vi "Result.vi"(8 "error in (no error)":errorcluster, 10 "Result":T1={"Case"="", "Message"="", "Description"="", "Status"=enum."Passed", "Result Type"=enum."Case", "Execution Time"=0.0}, 11 "Test Result Tree V2 in":refnum<class "Test Result Tree V2.lvclass">) -> (0 "error out":errorcluster, 3 "Test Result Tree V2 out":refnum<class "Test Result Tree V2.lvclass">)   [LabVIEW 2020, in "Test Result Tree V2.lvclass"]
uses:
  Test Result Tree V2.lvclass
  C:/Git/astemes-lunit/source/Framework/Helper Classes/Test Tree/Test Tree.lvclass
  Result/Result.ctl
  Result/Status.ctl
  Result/Type.ctl
  Test Tree/Test Tree.lvclass/Test Tree.ctl
  Utilities/Status to Glyph.vi
  Test Tree/Test Tree.lvclass
  Result/Result.lvlib
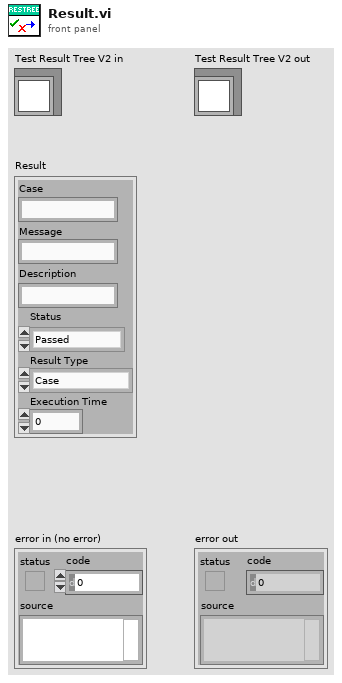
[diagram p1: front panel]
types:
  T1 = typedef "Result.lvlib/Result.ctl" = cluster{"Case":string, "Message":string, "Description":string, "Status":T2, "Result Type":T3, "Execution Time":dbl}
  T2 = typedef "Result.lvlib/Status.ctl" = enum16{"Passed", "Failed", "Error", "Skipped", "Setup Error", "Broken", "Teardown Error"}
  T3 = typedef "Result.lvlib/Type.ctl" = enum16{"Method", "Case", "Suite", "Pass", "Fail", "Skip", "Pass if", "Fail if", "Pass if Error", "Fail if Error", "Pass if Equal", "Fail if Equal"}
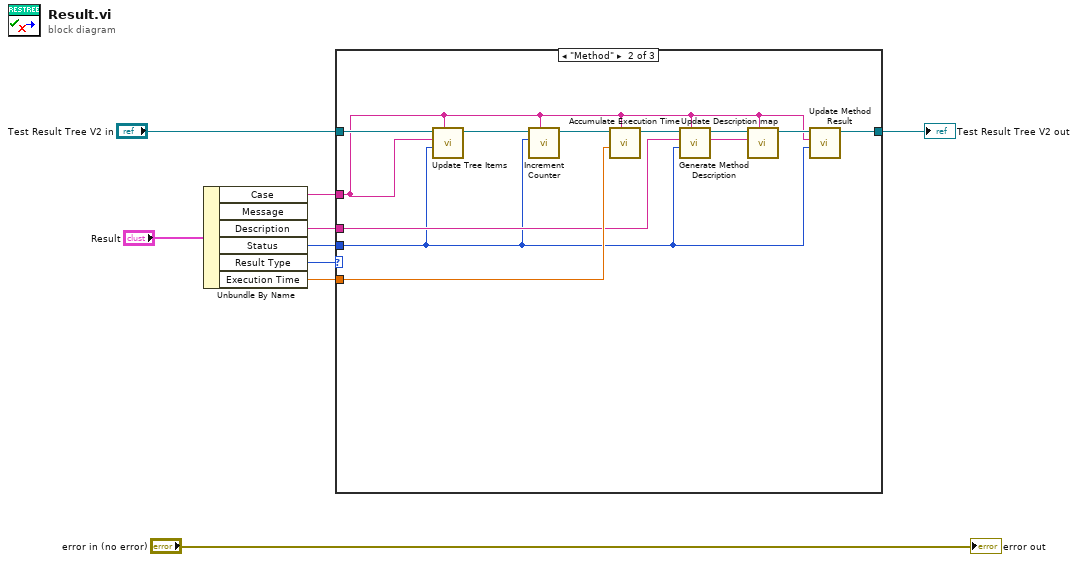
[diagram p0: block diagram]
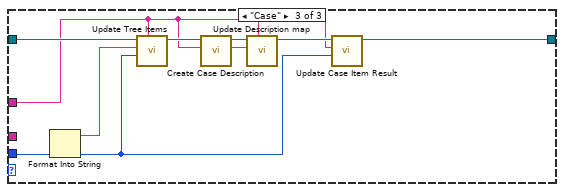
[diagram p3: hidden frame]
diagram:
  n1 = Unbundle By Name("Result") -> ("Case"=w5:string, "Description"=w1:string, "Status"=w4:T2, "Result Type"=w7:T3, "Execution Time"=w3:dbl)  [unwired: 1 out]
  n2 = case shown="\"Method\"" w7 {
    tunnel: "Test Result Tree V2 in" -> [w10 w20 w31]
    tunnel: [w10 w17 w25] -> w8
    tunnel: w5 -> [_ w12 w24]
    tunnel: w4 -> [_ w11 w23]
    tunnel: w3 -> [_ w19 _]
    tunnel: w1 -> [_ w13 _]
    frame Default {
    }
    frame "Method" {
      n3 = call "Update Tree Items.vi"("Item"=w12, "Status"=w11, "Child Text"=w12, "Test Tree In"=w20) -> ("Test Tree Out"=w21:refnum<class "Test Result Tree V2.lvclass">)  [unwired: 7 in]
      n4 = call "Increment Counter.vi"("Method Name"=w12, "Status"=w11, "Test Result Tree V2 in"=w21) -> ("Test Result Tree V2 out"=w22:refnum<class "Test Result Tree V2.lvclass">)  [unwired: 8 in]
      n5 = call "Accumulate Execution Time.vi"("Method Name"=w12, "Execution Time"=w19, "Test Result Tree V2 in"=w22) -> ("Test Result Tree V2 out"=w16:refnum<class "Test Result Tree V2.lvclass">)  [unwired: 8 in]
      n6 = call "Generate Method Description.vi"("Name"=w12, "Status"=w11, "Descirption"=w13, "Test Tree In"=w16) -> ("Description"=w14:string, "Test Tree Out"=w15:refnum<class "Test Result Tree V2.lvclass">)  [unwired: 6 in]
      n7 = call "Update Description map.vi"("Item"=w12, "Description"=w14, "Test Tree In"=w15) -> ("Test Tree Out"=w18:refnum<class "Test Result Tree V2.lvclass">)  [unwired: 8 in]
      n8 = call "Update Method Result.vi"("Status"=w11, "Case"=w12, "Test Tree In"=w18) -> ("Test Tree Out"=w17:refnum<class "Test Result Tree V2.lvclass">)  [unwired: 8 in]
    }
    frame "Case" {
      n9 = Format Into String(w23) -> (resulting string=w30:string)  [unwired: 3 in, 1 out]
      n10 = call "Update Tree Items.vi"("Item"=w24, "Status"=w23, "Child Text"=w30, "Test Tree In"=w31) -> ("Test Tree Out"=w29:refnum<class "Test Result Tree V2.lvclass">)  [unwired: 7 in]
      n11 = call "Create Case Description.vi"("Case"=w24, "Test Result Tree V2 in"=w29) -> ("Description"=w27:string, "Test Result Tree V2 in 2"=w28:refnum<class "Test Result Tree V2.lvclass">)  [unwired: 8 in]
      n12 = call "Update Description map.vi"("Item"=w24, "Description"=w27, "Test Tree In"=w28) -> ("Test Tree Out"=w26:refnum<class "Test Result Tree V2.lvclass">)  [unwired: 8 in]
      n13 = call "Update Case Item Result.vi"("Status"=w23, "Test Case"=w24, "Test Result Tree V2 in"=w26) -> ("Test Result Tree V2 out"=w25:refnum<class "Test Result Tree V2.lvclass">)  [unwired: 8 in]
    }
  }
  "Test Result Tree V2 out" <- w8
  "error out" <- "error in (no error)"
